vi "Begin.vi"(8 "error in":errorcluster) -> (0 "error out":errorcluster)   [LabVIEW 2014]
doc: "Called before other user functions, this VI is expected to open initial I/O refnums, load in file data, and do all program initialization. Notice that the <B>error out</B> terminal is simply used for data flow. Wiring it to other structures or subVIs ensures that this VI runs first."
uses:
  <vilib>/Rock Robotics/WPI/DriverStation/WPI_DriverStationRobotMode2.ctl
  <vilib>/Rock Robotics/SystemInterfaces/DIO/FPGA_DIOPWMChannel.ctl
  <vilib>/Rock Robotics/SystemInterfaces/DIO/FPGA_DIOChannel.ctl
  <vilib>/Rock Robotics/SystemInterfaces/AI/FPGA_AIChannel.ctl
  <vilib>/Rock Robotics/WPI/Joystick/WPI_JoystickDeviceEnum.ctl
  Variables/Default global.vi
  <vilib>/Rock Robotics/WPI/Compressor/WPI_CompressorGetSetRefNum.vi
  Variables/References.vi
  Navx_Library/navX-MXP Library/navX-MXP IMU.lvlib
panel:
  in  "error in 2":errorcluster
  out "error out 2":errorcluster
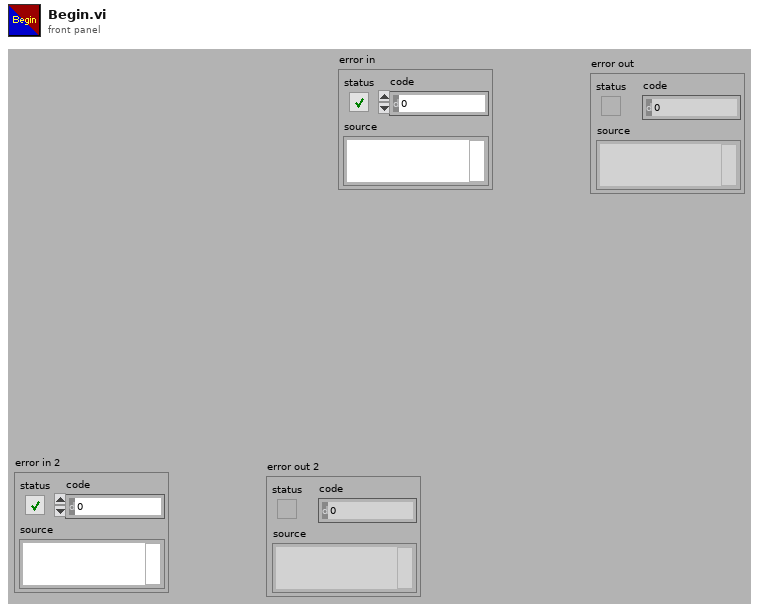
[diagram p1: front panel]
types:
  T1 = typedef "FPGA_DIOPWMChannel.ctl" = enum8{"PWM 0", "PWM 1", "PWM 2", "PWM 3", "PWM 4", "PWM 5", "PWM 6", "PWM 7", "PWM 8", "PWM 9", "PWM MXP 0", "PWM MXP 1", "PWM MXP 2", "PWM MXP 3", "PWM MXP 4", "PWM MXP 5", "PWM MXP 6", "PWM MXP 7", "PWM MXP 8", "PWM MXP 9", "Invalid"}
  T2 = typedef "FPGA_AIChannel.ctl" = enum8{"AI 0", "AI 1", "AI 2", "AI 3", "AI MXP 0", "AI MXP 1", "AI MXP 2", "AI MXP 3", "Invalid"}
  T3 = cluster{"Use CAN Turret?":bool, "PWM Channel Turret":T1, "Turret Encoder Location":enum16{"RoboRio", "Drive SRX", "Turret SRX"}, "CAN Device Number Turret":u8, "Turret Encoder Analog Channel":T2}
  T4 = typedef "FPGA_DIOChannel.ctl" = enum8{"DIO 0", "DIO 1", "DIO 2", "DIO 3", "DIO 4", "DIO 5", "DIO 6", "DIO 7", "DIO 8", "DIO 9", "DIO MXP 0", "DIO MXP 1", "DIO MXP 2", "DIO MXP 3", "DIO MXP 4", "DIO MXP 5", "DIO MXP 6", "DIO MXP 7", "DIO MXP 8", "DIO MXP 9", "DIO MXP 10", "DIO MXP 11", "DIO MXP 12", "DIO MXP 13", "DIO MXP 14", "DIO MXP 15", "Invalid"}
  T5 = cluster{"Use CAN Drive?":bool, "PWM Channel Drive":T1, "Drive Encoder Location":enum16{"RoboRio", "Drive SRX", "Turret SRX"}, "CAN Device Number Drive":u8, "RoboRIO Encoder":cluster{"Drive Encoder A Channel":T4, "Drive Encoder B Channel":T4}}
  T6 = typedef "WPI_DriverStationRobotMode2.ctl" = enum16{"Autonomous Disabled", "Autonomous Enabled", "Teleop Disabled", "Teleop Enabled", "Disconnected", "Finish", "Test Disabled", "Test Enabled", "Emergency Stopped"}
  T7 = typedef "WPI_CompressorDevRef.ctl" = cluster{"DevStatus":errorcluster, "Pneumatics Control Module":u8}
  T8 = typedef "WPI_JoystickDeviceEnum.ctl" = enum16{"USB 0", "USB 1", "USB 2", "USB 3", "USB 4", "USB 5"}
  T9 = typedef "WPI_JoystickDevRef.ctl" = cluster{"Device":T8}
  T10 = typedef "navX-MXP IMU.lvlib/navX Device TypeDef.ctl" = cluster{"navX Interface Protocol":T11, "navX Interface Protocol TypeDefs":cluster{"SPIDevRef":T12, "I2CDevRef":T15}, "navX System Information":cluster{"Board Information":T17, "Status":T18, "Offsets":T22}, "navX Common Information":cluster{"Update Rate (4Hz-60Hz)":T23, "refnum name":string, "error":errorcluster}}
  T11 = typedef "navX-MXP IMU.lvlib/navX Interface Protocol.ctl" = enum16{"SPI", "I2C"}
  T12 = typedef "WPI_SPIDevRef.ctl" = cluster{"DevStatus":errorcluster, "Handle":i32, "Controller":T13, "SPI Bus":T14}
  T13 = typedef "FPGA_TypedefDigitalModule.ctl" = enum16{"Controller 1"}
  T14 = typedef "spi_bus.ctl" = enum16{"SPI On-Board, CS0", "SPI On-Board, CS1", "SPI On-Board, CS2", "SPI On-Board, CS3", "SPI MXP", "Invalid"}
  T15 = typedef "WPI_I2CDevRef.ctl" = cluster{"DevStatus":errorcluster, "Controller":T13, "Device Address":u8, "Handle":i32, "I2C Bus":T16}
  T16 = typedef "i2c_bus.ctl" = enum16{"I2C On-Board", "I2C MXP", "Invalid"}
  T17 = typedef "navX-MXP IMU.lvlib/navX Board Information.ctl" = cluster{"WhoAmI (50 | 0x32)":u8, "Board Revision":u8, "Firmware Major Version":u8, "Firmware Minor Version":u8}
  T18 = typedef "navX-MXP IMU.lvlib/navX Status Data.ctl" = cluster{"Update Rate Hz":u8, "Accelerometer Full-Scale Range":u8, "Gyro Full-Scale Range":u16, "NAVX_OP_STATUS":T19, "NAVX_CAL_STATUS":T20, "NAVX_SELFTEST_STATUS":u8, "NAVX_SENSOR_STATUS":T21}
  T19 = typedef "navX-MXP IMU.lvlib/navX NAVX_OP_STATUS.ctl" = u8
  T20 = typedef "navX-MXP IMU.lvlib/navX NAVX_CAL_STATUS.ctl" = u8
  T21 = typedef "navX-MXP IMU.lvlib/navX NAVX_SENSOR_STATUS.ctl" = cluster{"MOVING":bool, "YAW_STABLE":bool, "MAG_DISTURBANCE":bool, "ALTITUDE_VALID":bool, "SEALEVEL_PRESS_SET":bool, "FUSED_HEADING_VALID":bool}
  T22 = typedef "navX-MXP IMU.lvlib/navX Offsets Data.ctl" = cluster{"Yaw":dbl, "Quat W":dbl, "Quat X":dbl, "Quat Y":dbl, "Quat Z":dbl}
  T23 = typedef "navX-MXP IMU.lvlib/navX Update Rate.ctl" = u8
  T24 = typedef "WPI_MotorControlDeviceRef.ctl" = cluster{"DeviceStatus":errorcluster, "Type":T25, "PWM":cluster{"Controller":T13, "PWM Channel":T1, "DeadBand":T26}, "CAN":cluster{"Device Number":u8, "Control Mode":T27, "Semaphore":T28, "Max Vout":dbl, "TalonSRX Control Mode":T29}, "Invert":bool, "TransformRef":T30, "InvTransformRef":T30}
  T25 = typedef "WPI_MotorControlType.ctl" = enum16{"PWM", "CAN", "CANTalonSRX"}
  T26 = typedef "WPI_PWMDeadband.ctl" = cluster{"Name":string, "maxPositivePwm":i32, "minPositivePwm":i32, "centerPwm":i32, "maxNegativePwm":i32, "minNegativePwm":i32, "angularRange":u16}
  T27 = typedef "WPI_CANJaguar_ControlMode.ctl" = enum8{"Percent VBus", "Current", "Speed", "Position", "Voltage"}
  T28 = typedef "Semaphore RefNum" = refnum<k1>
  T29 = typedef "WPI_CANTalonSRX_APIControlMode.ctl" = enum8{"Percent VBus", "Speed", "Position", "Slave", "Unchanged / Invalid"}
  T30 = typedef "WPI_PWMTransform_ConPane.ctl" = refnum<vi>
  T31 = typedef "WPI_AnalogChannelDevRef.ctl" = cluster{"DevStatus":errorcluster, "Controller":T32, "Analog Channel":T2}
  T32 = typedef "FPGA_TypedefAnalogModule.ctl" = enum16{"Controller 1"}
  T33 = typedef "WPI_EncoderDevRef.ctl" = cluster{"DevStatus":errorcluster, "EncoderIndex":T34, "CounterIndex":T35, "DistancePerCount":dbl, "Decoding Type":T36}
  T34 = typedef "FPGA_EncoderIdx.ctl" = enum8{"Enc 0", "Enc 1", "Enc 2", "Enc 3", "Enc 4", "Enc 5", "Enc 6", "Enc 7", "Invalid"}
  T35 = typedef "FPGA_CounterCtrSystemIndex.ctl" = enum8{"Ctr 0", "Ctr 1", "Ctr 2", "Ctr 3", "Ctr 4", "Ctr 5", "Ctr 6", "Ctr 7", "Invalid"}
  T36 = typedef "WPI_EncoderType.ctl" = enum16{"1x", "2x", "4x"}
  T37 = cluster{"DriveMotorRef":T24, "TurretMotorRef":T24, "Turret Encoder":cluster{"AIDeviceRef":T31, "Turret Analog Location":enum16{"RoboRio", "Drive SRX", "Turret SRX"}}, "Drive Encoder":cluster{"EncoderDevRef":T33, "Drive Encoder Location":enum16{"RoboRio", "Drive SRX", "Turret SRX"}}, "Pod position (RCS)":cluster{"X":dbl, "Y":dbl, "Z":dbl}, "Data":cluster{"Drive Motor Output":dbl, "Turret Motor Output":dbl, "Wheel RPM":dbl, "Turret Angle":dbl, "Turret angle offset":dbl, "Transmission moment of inertia":dbl, "Transmission efficiency":dbl, "Wheel dist / rev":dbl, "Turret moment of inertia":dbl, "Inv. turret encoder":bool, "Inv. drive encoder":bool}}
  T38 = cluster{"DriveMotorRef":T24, "TurretMotorRef":T24, "Turret Encoder":cluster{"AIDeviceRef":T31, "Turret Analog Location":enum16{"RoboRio", "Drive SRX", "Turret SRX"}}, "Drive Encoder":cluster{"EncoderDevRef":T33, "Drive Encoder Location":enum16{"RoboRio", "Drive SRX", "Turret SRX"}}, "Pod position (RCS)":cluster{"X":dbl, "Y":dbl, "Z":dbl}, "Data":cluster{"Drive Motor Output":dbl, "Turret Motor Output":dbl, "Wheel RPM":dbl, "Turret Angle":dbl, "Turret angle offset":dbl, "Transmission moment of inertia":dbl, "Transmission efficiency":dbl, "Wheel dist / rev":dbl, "Turret moment of inertia":dbl, "Inv. turret encoder":bool, "Inv. drive encoder":bool}}[]
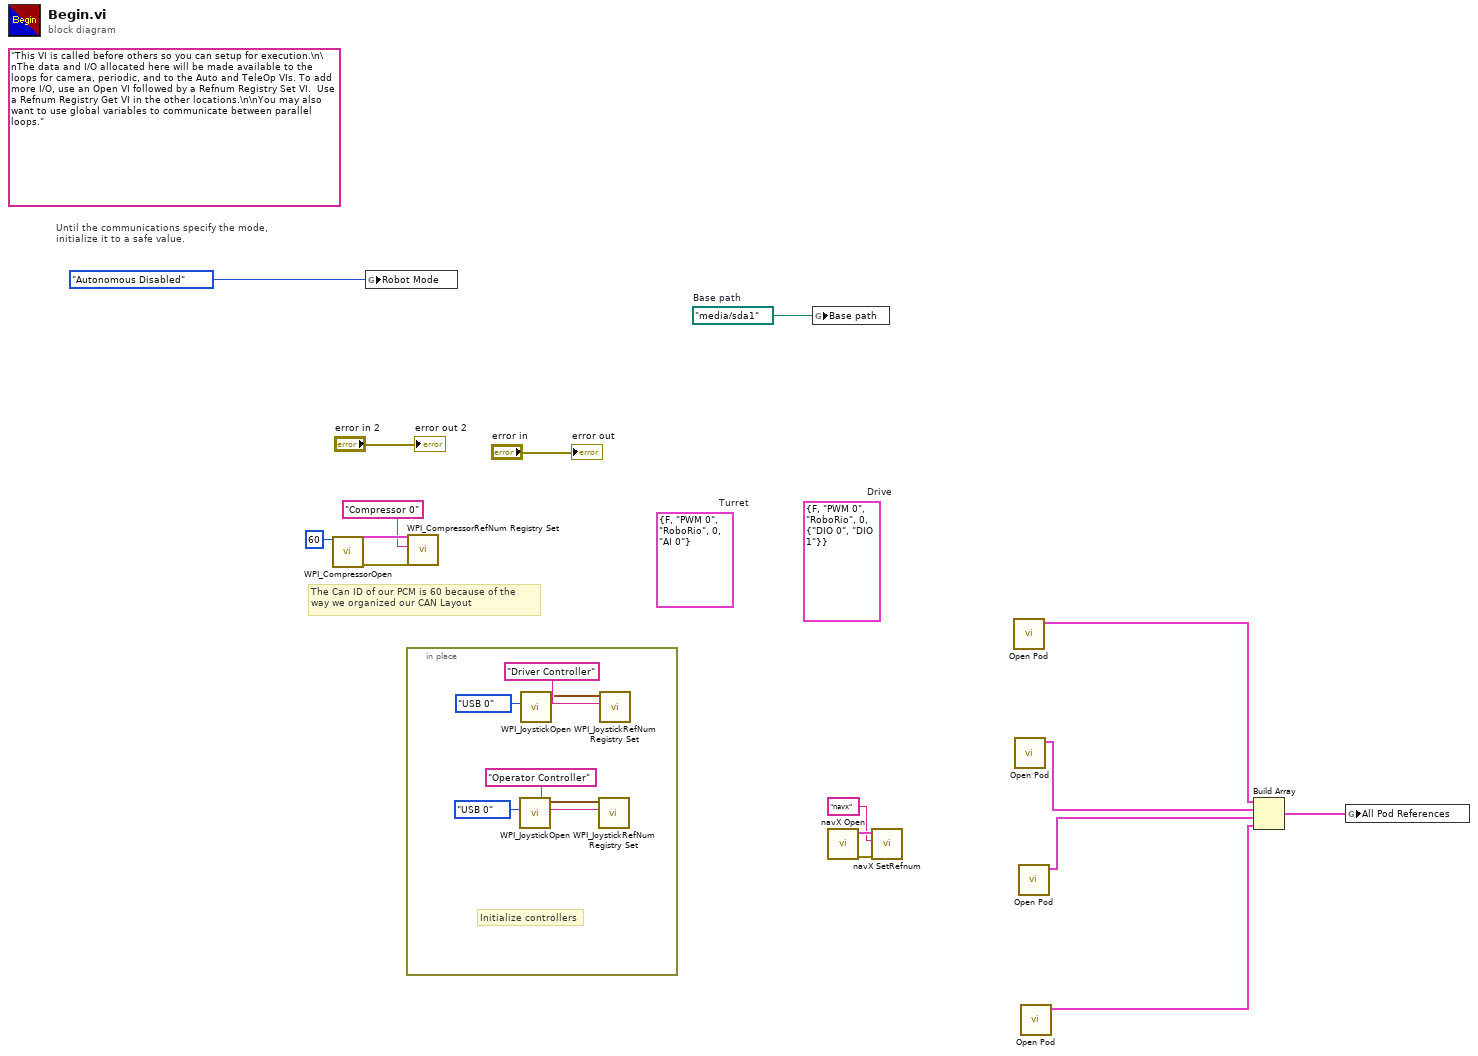
[diagram p0: block diagram]
diagram:
  w1 = path "/media/sda1"  # Base path
  (unwired) T3 {"Use CAN Turret?"=FALSE, "PWM Channel Turret"=enum."PWM 0", "Turret Encoder Location"=enum."RoboRio", "CAN Device Number Turret"=0, "Turret Encoder Analog Channel"=enum."AI 0"}  # Turret
  (unwired) T5 {"Use CAN Drive?"=FALSE, "PWM Channel Drive"=enum."PWM 0", "Drive Encoder Location"=enum."RoboRio", "CAN Device Number Drive"=0, "RoboRIO Encoder"={"Drive Encoder A Channel"=enum."DIO 0", "Drive Encoder B Channel"=enum."DIO 1"}}  # Drive
  (unwired) "This VI is called before others so you can setup for execution.\n\nThe data and I/O allocated here will be made available to the loops for camera, periodic, and to the Auto and TeleOp VIs. To add more I/O, use an Open VI followed by a Refnum Registry Set VI.  Use a Refnum Registry Get VI in the other locations.\n\nYou may also want to use global variables to communicate between parallel loops."
  # "The Can ID of our PCM is 60 because of the\nway we organized our CAN Layout"
  # "Until the communications specify the mode,\ninitialize it to a safe value."
  n1 = call <vilib>:"WPI_CompressorOpen.vi"("Pneumatics Control Module (0)"=u8 60) -> ("CompressorDevRef"=w13:T7, "error out"=w11:errorcluster)  [unwired: 13 in]
  n2 = global write "Default global.vi" "Robot Mode"(WPI_DriverStationRobotMode2."Autonomous Disabled" ("Robot Mode")) -> ()
  n3 = in-place {
    # "Initialize controllers"
    n4 = call <vilib>:"WPI_JoystickOpen.vi"("JoystickDevice"=WPI_JoystickDeviceEnum."USB 0") -> ("JoystickDevRef"=w18:T9)  [unwired: 10 in]
    n5 = call <vilib>:"WPI_JoystickOpen.vi"("JoystickDevice"=WPI_JoystickDeviceEnum."USB 0") -> ("JoystickDevRef"=w21:T9)  [unwired: 10 in]
    n6 = call <vilib>:"WPI_JoystickRefNum Registry Set.vi"("refnum name"="Operator Controller", "JoystickDevRef"=w18) -> ()  [unwired: 8 in, 2 out]
    n7 = call <vilib>:"WPI_JoystickRefNum Registry Set.vi"("refnum name"="Driver Controller", "JoystickDevRef"=w21) -> ()  [unwired: 8 in, 2 out]
  }
  n8 = call <vilib>:"WPI_CompressorRefNum Registry Set.vi"("error in (no error)"=w11, "refnum name"="Compressor 0", "CompressorDevRef"=w13) -> ()  [unwired: 7 in, 2 out]
  n9 = global write "Default global.vi" "Base path"(w1) -> ()
  n10 = call "navX Open.vi"() -> ("error out"=w3:errorcluster, "navX Device TypeDef"=w4:T10)  [unwired: 9 in, 1 out]
  n11 = call "navX SetRefnum.vi"("error in (no error)"=w3, "refnum name"="navx", "navX Device TypeDef"=w4) -> ()  [unwired: 7 in, 2 out]
  n12 = call "Open Pod.vi"() -> ("Pod and Turret"=w9:T37)  [unwired: 11 in]
  n13 = call "Open Pod.vi"() -> ("Pod and Turret"=w8:T37)  [unwired: 11 in]
  n14 = call "Open Pod.vi"() -> ("Pod and Turret"=w6:T37)  [unwired: 11 in]
  n15 = call "Open Pod.vi"() -> ("Pod and Turret"=w7:T37)  [unwired: 11 in]
  n16 = Build Array(w9, w8, w6, w7) -> (w5:T38)
  n17 = global write "References.vi" "All Pod References"(w5) -> ()
  "error out" <- "error in"
  "error out 2" <- "error in 2"
